vi "Diff_Drive_System_Acquire.vi"(6 "FPGA_Time_Seconds":dbl, 11 "DiffDriveDeviceRefs":T1 {"GyroDevRef"."Sample Rate" min=0.25 max=100.0 step=0.25}) -> (2 "Right Speed":dbl, 3 "Left Speed":dbl)   [LabVIEW 2019]
uses:
  <vilib>/Rock Robotics/WPI/Gyro/WPI_GyroDevRef.ctl
  <vilib>/Rock Robotics/SystemInterfaces/AI/FPGA_AIChannel.ctl
  <vilib>/Rock Robotics/SystemInterfaces/spilib/spi_bus.ctl
  <vilib>/Rock Robotics/WPI/Encoder/WPI_EncoderDevRef.ctl
  <vilib>/Rock Robotics/SystemInterfaces/Encoder/FPGA_EncoderIdx.ctl
  <vilib>/Rock Robotics/SystemInterfaces/Counter/FPGA_CounterCtrSystemIndex.ctl
  <vilib>/Rock Robotics/WPI/Encoder/WPI_EncoderType.ctl
  Diff_Drive_System_Globals.vi
  <vilib>/Rock Robotics/SystemInterfaces/DIO/FPGA_DIOPWMChannel.ctl
  <vilib>/Rock Robotics/WPI/PWM/WPI_PWMDeadband.ctl
  <vilib>/Rock Robotics/WPI/MotorControl/WPI_MotorControlType.ctl
  <vilib>/Rock Robotics/SystemInterfaces/DIO/FPGA_DIOChannel.ctl
  <vilib>/Rock Robotics/WPI/MotorControl/WPI_MotorControlDeviceRef.ctl
  <vilib>/Rock Robotics/WPI/RobotDrive/WPI_RobotDriveDevRef.ctl
  Diff_Drive_System_Device_Refs.ctl
panel:
  # "Analog"
  # "XRS"
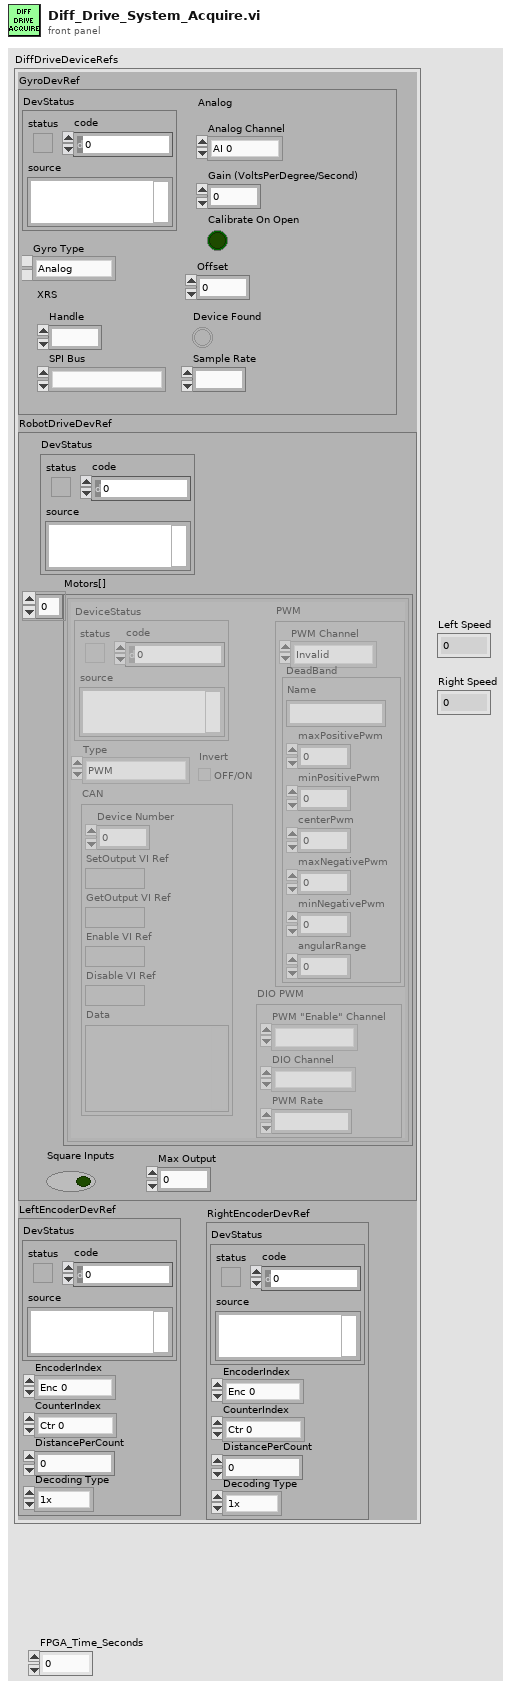
[diagram p1: front panel]
types:
  T1 = typedef "Diff_Drive_System_Device_Refs.ctl" = cluster{"GyroDevRef":T2, "RobotDriveDevRef":T5, "LeftEncoderDevRef":T11, "RightEncoderDevRef":T11}
  T2 = typedef "WPI_GyroDevRef.ctl" = cluster{"DevStatus":errorcluster, "Analog Channel":T3, "Gain (VoltsPerDegree/Second)":dbl, "Gyro Type":enum16{"Analog", "XRS450"}, "Handle":i32, "SPI Bus":T4, "Device Found":bool, "Sample Rate":dbl, "Calibrate On Open":bool, "Offset":dbl}
  T3 = typedef "FPGA_AIChannel.ctl" = enum8{"AI 0", "AI 1", "AI 2", "AI 3", "AI MXP 0", "AI MXP 1", "AI MXP 2", "AI MXP 3", "Invalid"}
  T4 = typedef "spi_bus.ctl" = enum16{"SPI On-Board, CS0", "SPI On-Board, CS1", "SPI On-Board, CS2", "SPI On-Board, CS3", "SPI MXP", "Invalid"}
  T5 = typedef "WPI_RobotDriveDevRef.ctl" = cluster{"DevStatus":errorcluster, "Motors[]":T6[], "Square Inputs":bool, "Max Output":dbl}
  T6 = typedef "WPI_MotorControlDeviceRef.ctl" = cluster{"DeviceStatus":errorcluster, "Type":T7, "PWM":cluster{"PWM Channel":T8, "DeadBand":T9}, "CAN":cluster{"Device Number":u8, "SetOutput VI Ref":variant, "GetOutput VI Ref":variant, "Enable VI Ref":variant, "Disable VI Ref":variant, "Data":variant}, "Invert":bool, "DIO PWM":cluster{"PWM \"Enable\" Channel":T8, "DIOChannel":T10, "PWM Rate":dbl}}
  T7 = typedef "WPI_MotorControlType.ctl" = enum16{"PWM", "CAN", "DIO PWM"}
  T8 = typedef "FPGA_DIOPWMChannel.ctl" = enum8{"PWM 0", "PWM 1", "PWM 2", "PWM 3", "PWM 4", "PWM 5", "PWM 6", "PWM 7", "PWM 8", "PWM 9", "PWM MXP 0", "PWM MXP 1", "PWM MXP 2", "PWM MXP 3", "PWM MXP 4", "PWM MXP 5", "PWM MXP 6", "PWM MXP 7", "PWM MXP 8", "PWM MXP 9", "Invalid"}
  T9 = typedef "WPI_PWMDeadband.ctl" = cluster{"Name":string, "maxPositivePwm":i32, "minPositivePwm":i32, "centerPwm":i32, "maxNegativePwm":i32, "minNegativePwm":i32, "angularRange":u16}
  T10 = typedef "FPGA_DIOChannel.ctl" = enum8{"DIO 0", "DIO 1", "DIO 2", "DIO 3", "DIO 4", "DIO 5", "DIO 6", "DIO 7", "DIO 8", "DIO 9", "DIO MXP 0", "DIO MXP 1", "DIO MXP 2", "DIO MXP 3", "DIO MXP 4", "DIO MXP 5", "DIO MXP 6", "DIO MXP 7", "DIO MXP 8", "DIO MXP 9", "DIO MXP 10", "DIO MXP 11", "DIO MXP 12", "DIO MXP 13", "DIO MXP 14", "DIO MXP 15", "SPI Port CS1", "SPI Port CS2", "SPI Port CS3", "SPI Port MISO", "SPI Port MOSI", "Invalid"}
  T11 = typedef "WPI_EncoderDevRef.ctl" = cluster{"DevStatus":errorcluster, "EncoderIndex":T12, "CounterIndex":T13, "DistancePerCount":dbl, "Decoding Type":T14}
  T12 = typedef "FPGA_EncoderIdx.ctl" = enum8{"Enc 0", "Enc 1", "Enc 2", "Enc 3", "Enc 4", "Enc 5", "Enc 6", "Enc 7", "Invalid"}
  T13 = typedef "FPGA_CounterCtrSystemIndex.ctl" = enum8{"Ctr 0", "Ctr 1", "Ctr 2", "Ctr 3", "Ctr 4", "Ctr 5", "Ctr 6", "Ctr 7", "Invalid"}
  T14 = typedef "WPI_EncoderType.ctl" = enum16{"1x", "2x", "4x"}
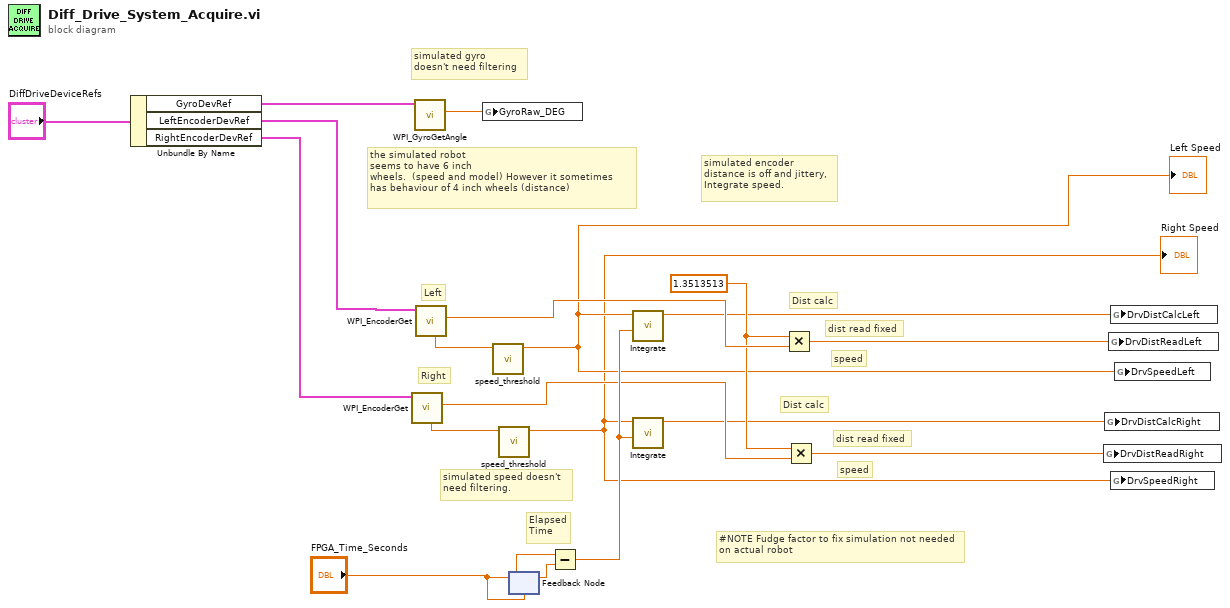
[diagram p0: block diagram]
diagram:
  w12 = 1.3513513
  # "#NOTE Fudge factor to fix simulation not needed on actual robot"
  # "Elapsed\nTime"
  # "simulated speed doesn't\nneed filtering."
  # "simulated gyro \ndoesn't need filtering"
  # "Right"
  # "Left"
  # "the simulated robot\nseems to have 6 inch\nwheels.  (speed and model) However it sometimes\nhas behaviour of 4 inch wheels (distance)"
  # "speed"
  # "dist read fixed"
  # "Dist calc"
  # "speed"
  # "dist read fixed"
  # "Dist calc"
  # "simulated encoder\ndistance is off and jittery,\nIntegrate speed."
  n1 = Unbundle By Name("DiffDriveDeviceRefs") -> ("GyroDevRef"=w3:T2, "LeftEncoderDevRef"=w2:T11, "RightEncoderDevRef"=w1:T11)
  n2 = call <vilib>:"WPI_EncoderGet.vi"("EncoderDevRef"=w1) -> ("Distance"=w14:dbl, "Rate"=w16:dbl)  [unwired: 5 in, 4 out]
  n3 = call <vilib>:"WPI_GyroGetAngle.vi"("GyroDevRef"=w3) -> ("Angle"=w11:dbl)  [unwired: 6 in, 4 out]
  n4 = call <vilib>:"WPI_EncoderGet.vi"("EncoderDevRef"=w2) -> ("Distance"=w13:dbl, "Rate"=w15:dbl)  [unwired: 5 in, 4 out]
  n5 = global write "Diff_Drive_System_Globals.vi" "GyroRaw_DEG"(w11) -> ()
  n6 = call "speed_threshold.vi"("SPEED IN"=w15) -> ("SPEED OUT"=w8:dbl)  [unwired: 10 in]
  "Left Speed" <- w8
  n7 = call "speed_threshold.vi"("SPEED IN"=w16) -> ("SPEED OUT"=w5:dbl)  [unwired: 10 in]
  "Right Speed" <- w5
  n8 = feedback #1("FPGA_Time_Seconds") -> (w17:dbl)
  n9 = feedback-in #1("FPGA_Time_Seconds") -> ()
  n10 = Subtract(x="FPGA_Time_Seconds", y=w17) -> (x-y=w18:dbl)
  n11 = call "Integrate.vi"("Elapsed Sec"=w18, "Rate"=w8) -> ("DIST"=w10:dbl)  [unwired: 9 in]
  n12 = call "Integrate.vi"("Elapsed Sec"=w18, "Rate"=w5) -> ("DIST"=w7:dbl)  [unwired: 9 in]
  n13 = Multiply(x=w12, y=w13) -> (x*y=w9:dbl)
  n14 = Multiply(x=w12, y=w14) -> (x*y=w6:dbl)
  n15 = global write "Diff_Drive_System_Globals.vi" "DrvDistReadRight"(w6) -> ()
  n16 = global write "Diff_Drive_System_Globals.vi" "DrvDistCalcRight"(w7) -> ()
  n17 = global write "Diff_Drive_System_Globals.vi" "DrvDistReadLeft"(w9) -> ()
  n18 = global write "Diff_Drive_System_Globals.vi" "DrvDistCalcLeft"(w10) -> ()
  n19 = global write "Diff_Drive_System_Globals.vi" "DrvSpeedRight"(w5) -> ()
  n20 = global write "Diff_Drive_System_Globals.vi" "DrvSpeedLeft"(w8) -> ()
